vi "OpenTcp.vi"   [LabVIEW 2018]
uses:
  <vilib>/Plasmionique/MB Master/MB_Master_TCP/MB_Master_TCP.lvclass
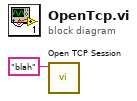
[diagram p0: block diagram]
diagram:
  n1 = call <vilib>:"Open TCP Session.vi"("IP Address"="blah") -> ()  [unwired: 9 in, 2 out]
